vi "Read Waveform (Single).vi"(6 "Timeout (10000 ms)":i32=10000 min=1, 8 "error in (no error)":errorcluster, 10 "Trace (0: U1)":i32(ring) items=["U1", "I1", "U2", "I2", "U3", "I3", "U4", "I4", "U5", "I5", "U6", "I6", "Speed", "Torque", "AUX1", "AUX2"], 11 "VISA resource name":refnum<visa-resource-name>) -> (0 "error out":errorcluster, 2 "Waveform Data":T1(graph), 3 "VISA resource name out":refnum<visa-resource-name>)   [LabVIEW 2021, in "Yokogawa WT1800 Series.lvlib"]
doc: "The VI waits for the acquisition to complete and returns the waveform of the trace you specified. If the insturument did not complete the acquisition within the time period you specify with the <b>Timeout</b> parameter, the VI returns a time out error. A common cause for a timeout error is the acquisition was not triggered. For example, the trigger level is out of range of the waveform.\n\nCall the <B>Fetch Waveform</B> VI to obtain the waveforms for each of the remaining enabled trace."
uses:
  <instrlib>/Yokogawa WT1800 Series/Yokogawa WT1800 Series.lvlib
panel:
  # "ms"
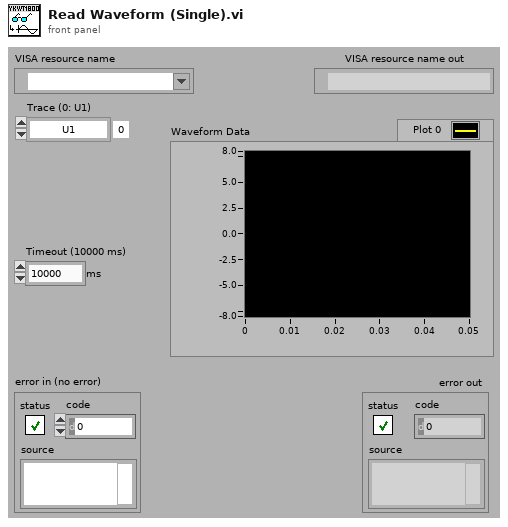
[diagram p1: front panel]
types:
  T1 = cluster{"start":dbl, "Sampling Time":dbl, "Output":dbl[]}
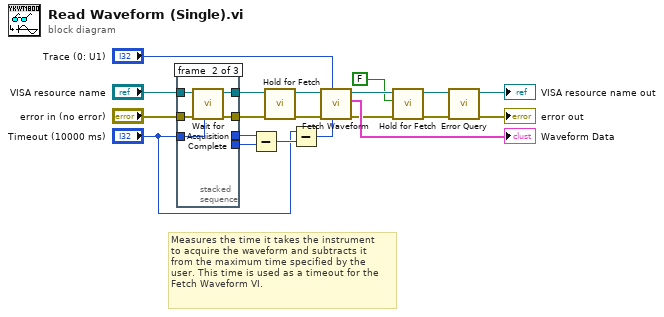
[diagram p0: block diagram]
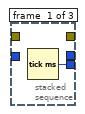
[diagram p2: hidden frame]
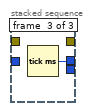
[diagram p3: hidden frame]
diagram:
  # "Measures the time it takes the instrument \nto acquire the waveform and subtracts it \nfrom the maximum time specified by the \nuser. This time is used as a timeout for the \nFetch Waveform VI."
  n1 = stacked-sequence {
    tunnel: "VISA resource name" -> [_ w25 _]
    tunnel: [_ w23 _] -> w9
    tunnel: "error in (no error)" -> [_ w24 _]
    tunnel: [_ w22 _] -> w7
    tunnel: [w21 _ _] -> w15
    tunnel: "Timeout (10000 ms)" -> [_ w26 _]
    tunnel: [_ _ w27] -> w13
    frame #0 {
      n2 = Tick Count (ms)() -> (millisecond timer value=w21:u32)
    }
    frame #1 {
      n3 = call <instrlib>:"Wait for Acquisition Complete.vi"("Timeout (10000 ms)"=w26, "error in (no error)"=w24, "VISA resource name"=w25) -> ("error out"=w22:errorcluster, "VISA resource name out"=w23:refnum<visa-resource-name>)  [unwired: 7 in]
    }
    frame #2 {
      n4 = Tick Count (ms)() -> (millisecond timer value=w27:u32)
    }
  }
  n5 = Subtract(x=w13, y=w15) -> (x-y=w17:u32)
  n6 = call <instrlib>:"Hold for Fetch.vi"("error in (no error)"=w7, "VISA resource name"=w9) -> ("error out"=w6:errorcluster, "VISA resource name out"=w8:refnum<visa-resource-name>)  [unwired: 8 in]
  n7 = Subtract(x="Timeout (10000 ms)", y=w17) -> (x-y=w16:u32)
  n8 = call <instrlib>:"Fetch Waveform.vi"("Timeout (10000 ms)"=w16, "Trace (0: U1)"="Trace (0: U1)", "error in (no error)"=w6, "VISA resource name"=w8) -> ("error out"=w3:errorcluster, "Waveform Data"=→"Waveform Data":T1, "VISA resource name out"=w5:refnum<visa-resource-name>)  [unwired: 5 in]
  n9 = call <instrlib>:"Hold for Fetch.vi"("error in (no error)"=w3, "Hold for Fetch (T: Enable)"=FALSE, "VISA resource name"=w5) -> ("error out"=w2:errorcluster, "VISA resource name out"=w4:refnum<visa-resource-name>)  [unwired: 7 in]
  n10 = call <instrlib>:"Error Query.vi"("error in (no error)"=w2, "VISA resource name"=w4) -> ("error out"=→"error out":errorcluster, "VISA resource name out"=→"VISA resource name out":refnum<visa-resource-name>)  [unwired: 6 in, 2 out]
